vi "DestroyTestSuite.vi"(8 "error in (no error)":errorcluster, 11 "Test Runner in":refnum<class "Test Runner.lvclass">) -> (0 "error out":errorcluster, 2 "Test Suite Results":refnum<class "Test Result.lvclass">, 3 "Test Runner out":refnum<class "Test Runner.lvclass">)   [LabVIEW 2013, in "Caraya.lvlib" / "Test Runner.lvclass"]
uses:
  Test Runner.lvclass
  Test Result/Test Result.lvclass
  Test Runner.lvclass/Test Runner.ctl
  Test Suite/Test Suite.lvclass
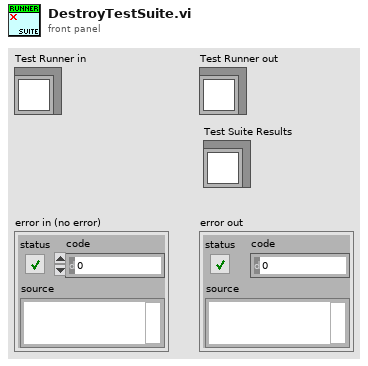
[diagram p1: front panel]
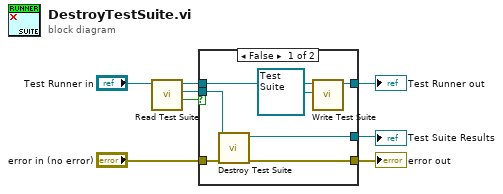
[diagram p0: block diagram]
diagram:
  n1 = call "Read Test Suite.vi"("Test Runner in"="Test Runner in") -> ("undefined"=w2:bool, "Test Suite"=w6:refnum<class "Test Suite.lvclass">, "Test Runner out"=w7:refnum<class "Test Runner.lvclass">)  [unwired: 8 in]
  n2 = case shown="False" w2 {
    tunnel: [w15 w16] -> w3
    tunnel: "error in (no error)" -> [w14 w16]
    tunnel: w6 -> [w13 _]
    tunnel: w7 -> [w12 w17]
    tunnel: [w11 w17] -> w8
    tunnel: [w9 _] -> w1
    frame False {
      n3 = call-dynamic "Destroy Test Suite.vi"("error in (no error)"=w14, "Test Suite in"=w13) -> ("error out"=w15:errorcluster, "Test Suite Results"=w9:refnum<class "Test Result.lvclass">)  [unwired: 8 in]
      n4 = call "Write Test Suite.vi"("Test Suite"=refnum<class "Test Suite.lvclass"> refnum, "Test Runner in"=w12) -> ("Test Runner out"=w11:refnum<class "Test Runner.lvclass">)  [unwired: 9 in]
    }
    frame True {
    }
  }
  "Test Runner out" <- w8
  "error out" <- w3
  "Test Suite Results" <- w1
